vi "SetRoi.vi"() -> ()   [LabVIEW 2011]
panel:
  in  "SetRoi":bool
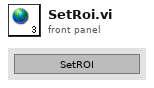
[diagram p1: front panel]
diagram:
